vi "topic.vi"(9 "Amount of topics":i32=5, 11 "project-param out 4":T1) -> (3 "project-param out 3":T1)   [LabVIEW 2019]
uses:
  Project Parameters.ctl
  <vilib>/numeric/Random Number (Range) I64.vi
  <vilib>/numeric/sub_Random U32.vi
panel:
  out "String":string
  out "array":string[](array[string])
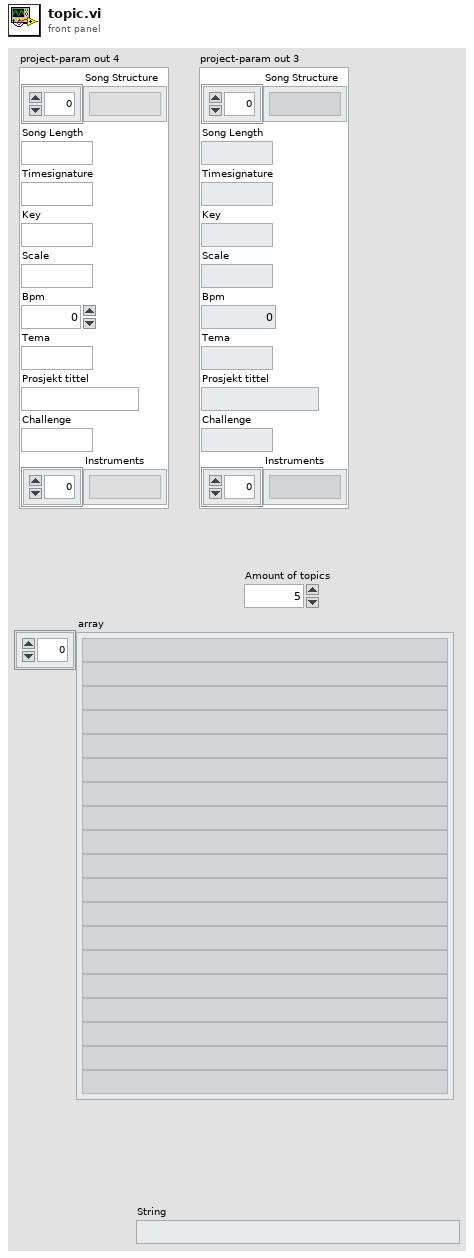
[diagram p1: front panel]
types:
  T1 = typedef "Project Parameters.ctl" = cluster{"Song Structure":string[], "Song Length":string, "Timesignature":string, "Key":string, "Scale":string, "Bpm":i32, "Tema":string, "Prosjekt tittel":string, "Challenge":string, "Instruments":string[]}
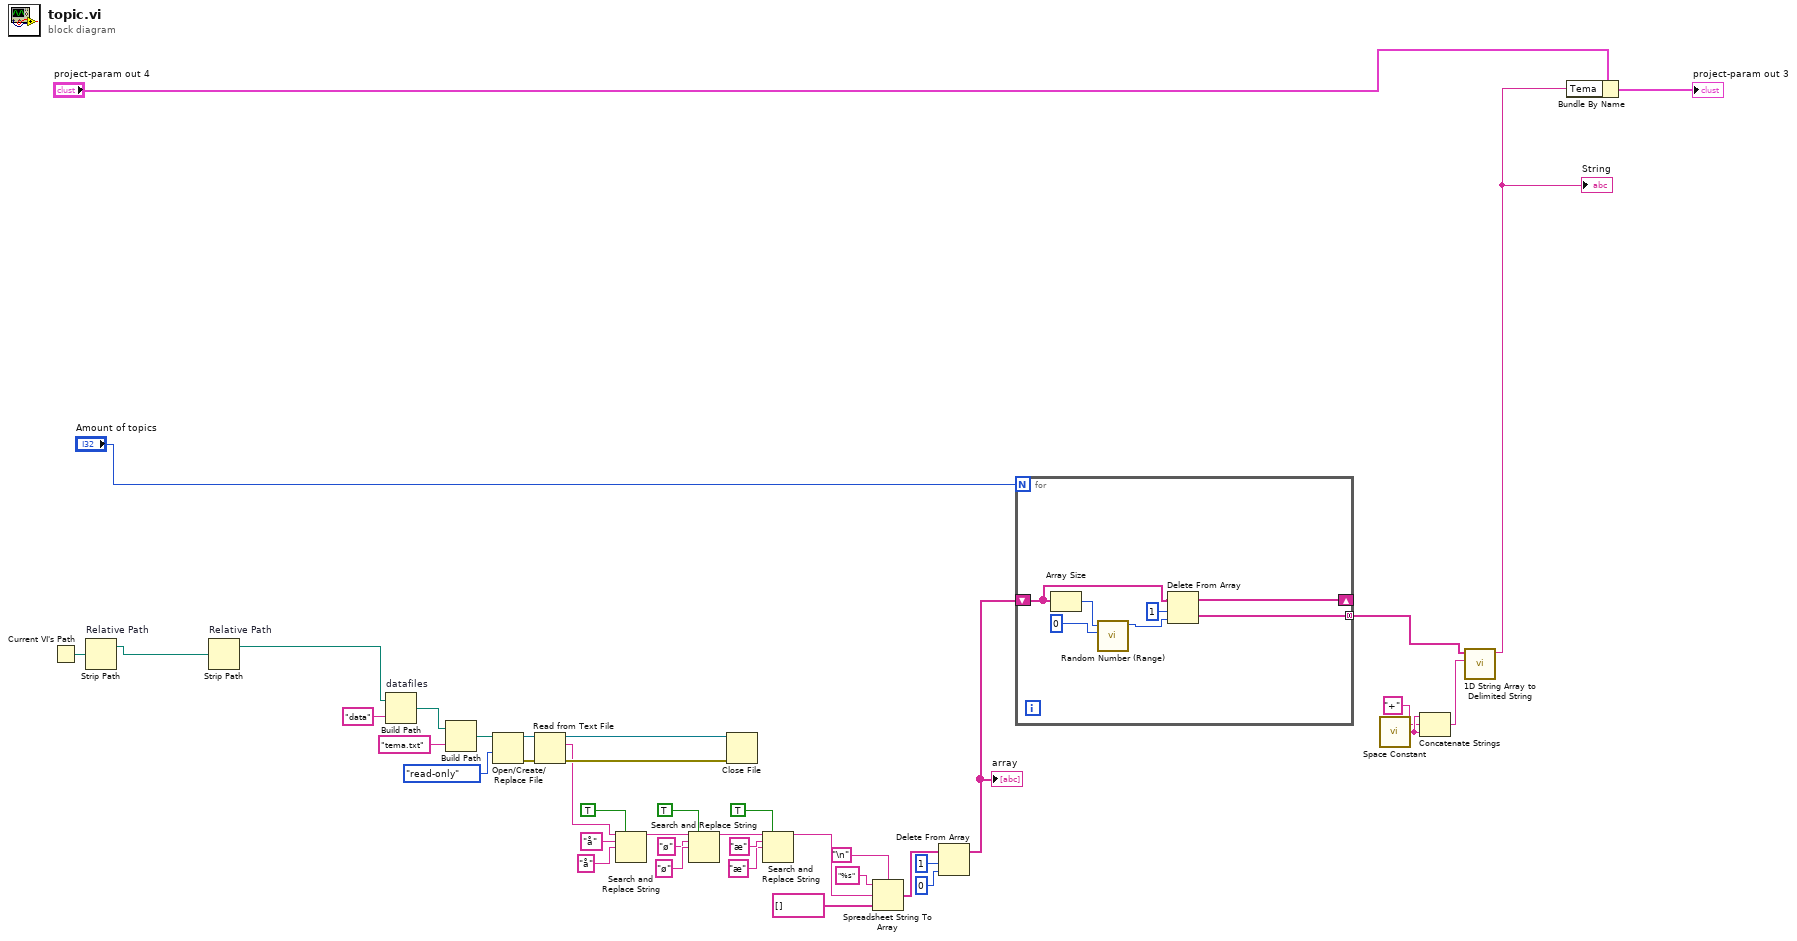
[diagram p0: block diagram]
diagram:
  n1 = Current VI's Path() -> (path=w38:path)
  n2 = Strip Path "Relative Path"(path=w38) -> (stripped path=w2:path)  [unwired: 1 out]
  n3 = Strip Path "Relative Path"(path=w2) -> (stripped path=w1:path)  [unwired: 1 out]
  n4 = Build Path "datafiles"(base path=w1, name or relative path="data") -> (appended path=w30:path)
  n5 = Build Path(base path=w30, name or relative path="tema.txt") -> (appended path=w29:path)
  n6 = Open/Create/Replace File(file path (use dialog)=w29, access (0:read/write)=enum16{"read/write", "read-only", "write-only"}."read-only") -> (refnum out=w35:refnum<file>, error out=w34:errorcluster)  [unwired: 4 in, 1 out]
  n7 = Read from Text File(file (use dialog)=w35, error in=w34) -> (refnum out=w33:refnum<file>, text=w25:string, error out=w32:errorcluster)  [unwired: 2 in, 1 out]
  n8 = Search and Replace String(replace all?=TRUE ("replace all? (F)"), input string=w25, search string="å", replace string="å" ("replace string (\"\")")) -> (result string=w18:string)  [unwired: 4 in, 3 out]
  n9 = Search and Replace String(replace all?=TRUE ("replace all? (F)"), input string=w18, search string="ø", replace string="ø" ("replace string (\"\")")) -> (result string=w14:string)  [unwired: 4 in, 3 out]
  n10 = Close File(refnum=w33, error in=w32) -> ()  [unwired: 2 out]
  n11 = Search and Replace String(replace all?=TRUE ("replace all? (F)"), input string=w14, search string="æ", replace string="æ" ("replace string (\"\")")) -> (result string=w13:string)  [unwired: 4 in, 3 out]
  n12 = Spreadsheet String To Array(delimiter (Tab)="\n", format string="%s", spreadsheet string=w13, array type (2D Dbl)=string[] []) -> (array=w12:string[])
  n13 = Delete From Array(array=w12, length=1, index=0) -> (array with subset deleted=w9:string[])  [unwired: 1 out]
  "array" <- w9
  n14 = for {
    N: "Amount of topics" -> [_]
    shift-right: [w42] -> _
    shift-left: w9 -> [w45]
    tunnel: [w41] -> w4 mode=concatenating
    n15 = Array Size(array=w45) -> (size(s)=w47:i32)
    n16 = call-poly <vilib>:"Random Number (Range).vi"("lower bound (-100)"=i64 0, "upper bound (100)"=w47) -> ("number"=w43:i64)  [unwired: 9 in]
    n17 = Delete From Array(array=w45, length=1, index=w43) -> (deleted portion=w41:string[], array with subset deleted=w42:string[])
  }
  n18 = call <vilib>:"Space Constant.vi"() -> ("String"=w6:string)
  n19 = Concatenate Strings(w6, "+" ("string"), w6) -> (w7:string)
  n20 = call <vilib>:"1D String Array to Delimited String.vi"("delimiter"=w7, "string array"=w4) -> ("delimited string"=w3:string)  [unwired: 9 in]
  "String" <- w3
  n21 = Bundle By Name(cluster="project-param out 4", "Tema"=w3) -> (→"project-param out 3":T1)
